vi "Teleop.vi"(10 "Match Info":T1={"Autonomous Elapsed Seconds"=0.0, "TeleOp Elapsed Seconds"=0.0, "Disabled Elapsed Seconds"=0.0, "Visited Autonomous"=FALSE, "Visited TeleOp"=FALSE, "Visited Disabled"=FALSE, "Autonomous Settings"={"Autonomous Style"=enum."Independent", "VI Refnum"=refnum}}, 11 "Call Context":T2) -> ()   [LabVIEW 2019]
doc: "This VI is called for each enabled TeleOp packet received from the DS. It is typically used to read from joysticks and other inputs and update I/O or setpoints for timed control loops. It should complete and return within 20 milliseconds or risk missing DS packets."
uses:
  <vilib>/Rock Robotics/WPI/DriverStation/WPI_DriverStationDerivedRobotMode.ctl
  <vilib>/Rock Robotics/WPI/DriverStation/WPI_DriverStationMatch Info.ctl
  Framework/Robot Global Data.vi
  <vilib>/Rock Robotics/Network Tables/NT Write Boolean.vi
  <vilib>/Rock Robotics/Network Tables/NT Write Number.vi
  <vilib>/Rock Robotics/Network Tables/NT Write Numeric Array.vi
  <vilib>/Rock Robotics/Network Tables/NT Write Boolean Array.vi
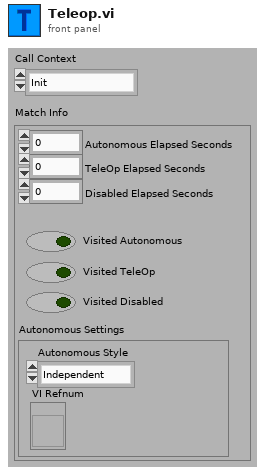
[diagram p1: front panel]
types:
  T1 = typedef "WPI_DriverStationMatch Info.ctl" = cluster{"Autonomous Elapsed Seconds":dbl, "TeleOp Elapsed Seconds":dbl, "Disabled Elapsed Seconds":dbl, "Visited Autonomous":bool, "Visited TeleOp":bool, "Visited Disabled":bool, "Autonomous Settings":cluster{"Autonomous Style":enum16{"Iterative", "Independent"}, "VI Refnum":refnum<vi>}}
  T2 = typedef "WPI_DriverStationDerivedRobotMode.ctl" = enum16{"Init", "Execute", "Stop"}
  T3 = typedef "WPI_JoystickDevRef.ctl" = cluster{"Device":T4}
  T4 = typedef "WPI_JoystickDeviceEnum.ctl" = enum16{"USB 0", "USB 1", "USB 2", "USB 3", "USB 4", "USB 5"}
  T5 = typedef "Command Status Info.ctl" = cluster{"Name":string, "Status":T6, "notifier out":T7}
  T6 = typedef "Completion Status.ctl" = enum16{"Successful", "Aborted", "Incomplete"}
  T7 = typedef "Completion Notifier.ctl" = refnum<notifier>
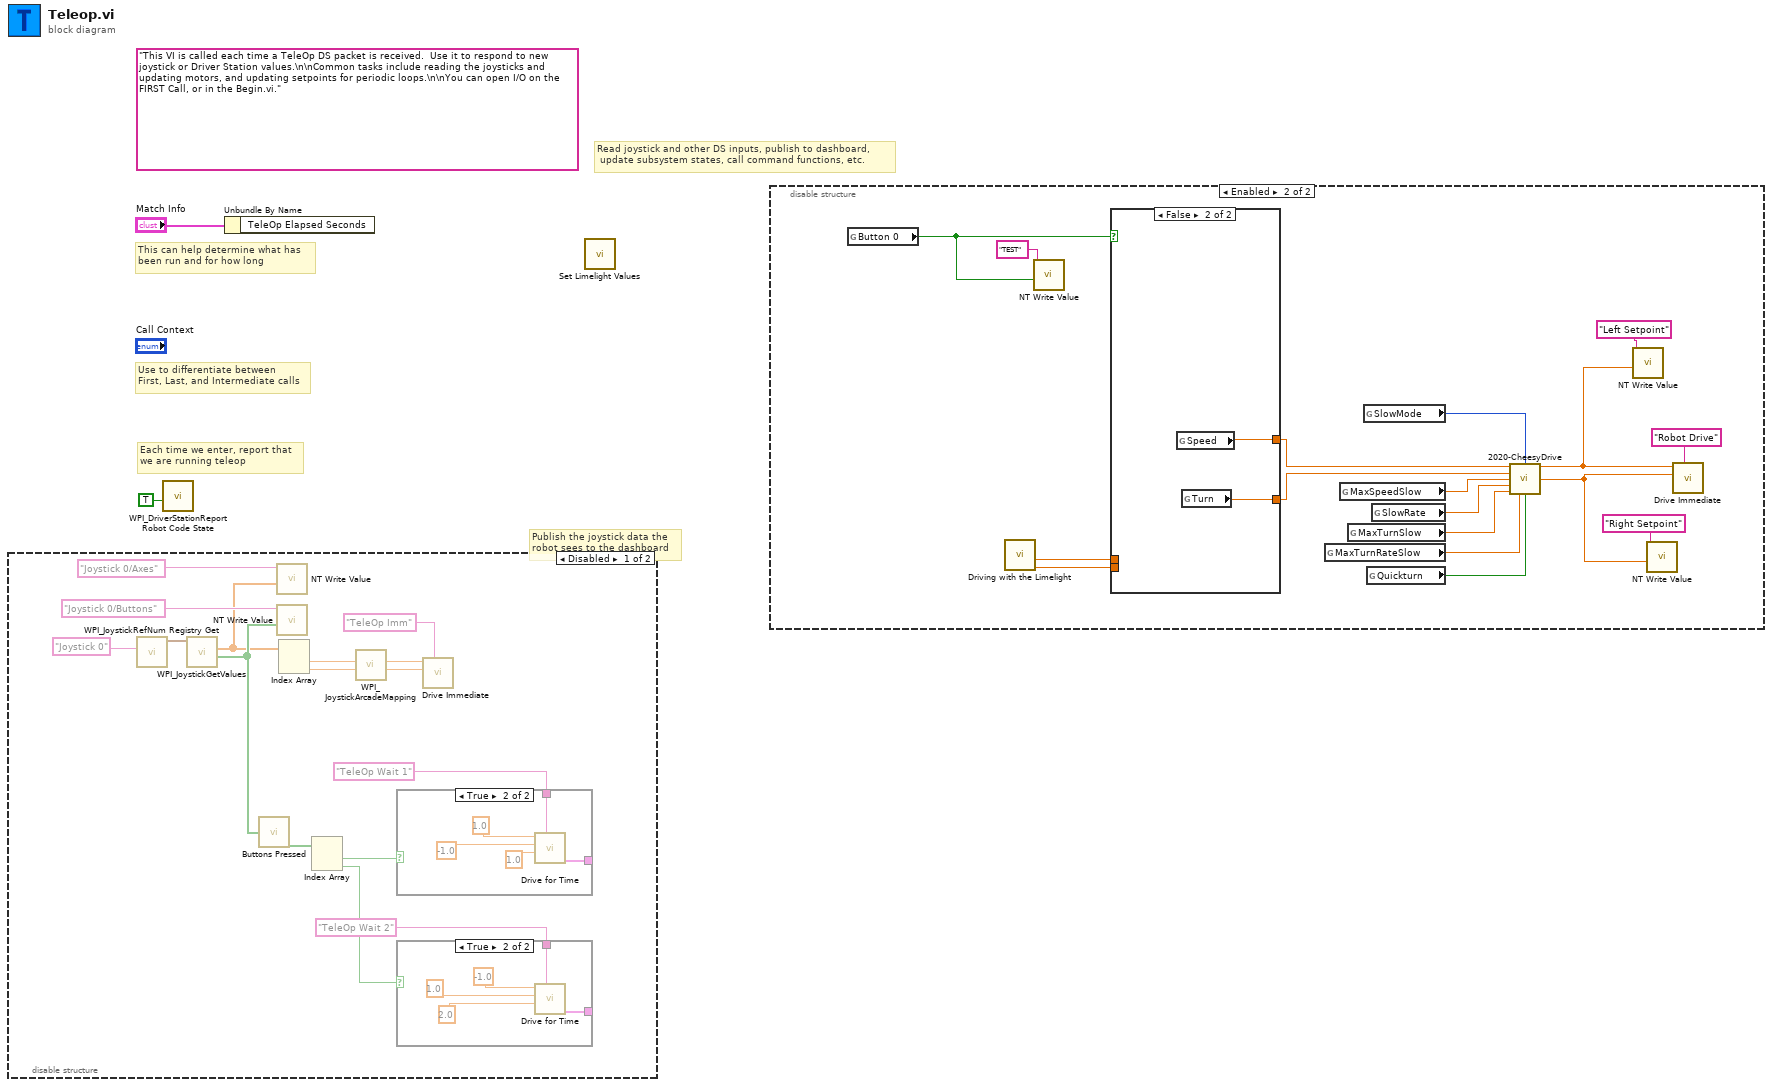
[diagram p0: block diagram]
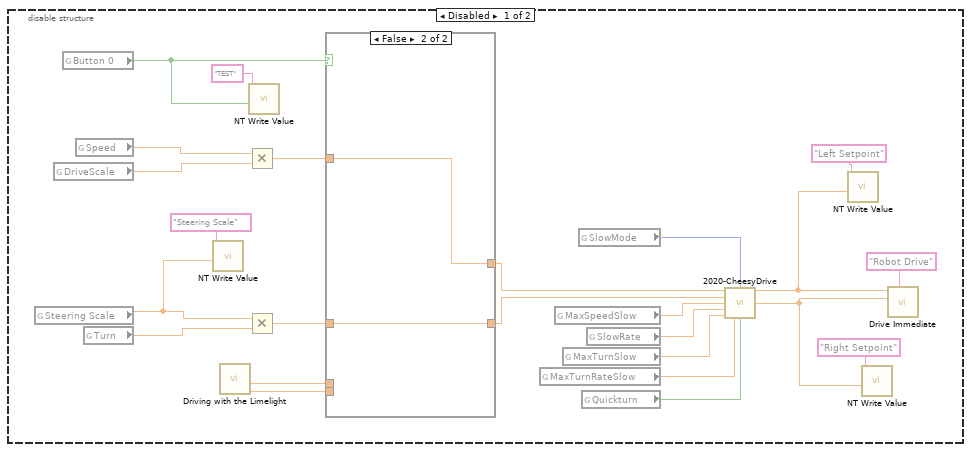
[diagram p2: hidden frame]
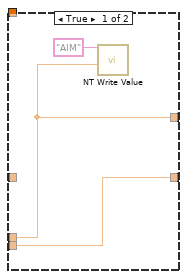
[diagram p3: hidden frame]
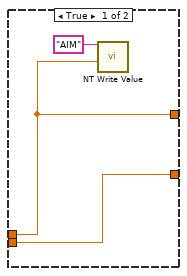
[diagram p4: hidden frame]
diagram:
  (unwired) "This VI is called each time a TeleOp DS packet is received.  Use it to respond to new joystick or Driver Station values.\n\nCommon tasks include reading the joysticks and updating motors, and updating setpoints for periodic loops.\n\nYou can open I/O on the FIRST Call, or in the Begin.vi."
  # "Publish the joystick data the\nrobot sees to the dashboard"
  # "Read joystick and other DS inputs, publish to dashboard,\n update subsystem states, call command functions, etc."
  # "Each time we enter, report that\nwe are running teleop"
  # "Use to differentiate between\nFirst, Last, and Intermediate calls"
  # "This can help determine what has\nbeen run and for how long"
  n1 = disable-structure shown="Disabled" {
    frame Disabled {
      n2 = call <vilib>:"WPI_JoystickRefNum Registry Get.vi"("refnum name"="Joystick 0") -> ("JoystickDevRef"=w17:T3)  [unwired: 1 in, 9 out]
      n3 = call <vilib>:"WPI_JoystickGetValues.vi"("JoystickDevRef"=w17) -> ("Buttons"=w5:bool[], "Axes"=w4:dbl[])  [unwired: 6 in, 3 out]
      n4 = call "Buttons Pressed.vi"("Button Values"=w5) -> ("Button Presses"=w13:bool[])
      n5 = call-poly <vilib>:"NT Write Value.vi"("Numeric Array"=w4, "Name"="Joystick 0/Axes") -> ()  [unwired: 9 in, 1 out]
      n6 = call-poly <vilib>:"NT Write Value.vi"("Boolean Array"=w5, "Name"="Joystick 0/Buttons") -> ()  [unwired: 9 in, 1 out]
      n7 = Index Array(array=w4) -> (element #1=w8:dbl, element #2=w7:dbl)  [unwired: 2 in]
      n8 = Index Array(array=w13) -> (element #1=w12:bool, element #2=w11:bool)  [unwired: 2 in]
      n9 = call <vilib>:"WPI_JoystickArcadeMapping.vi"("Y axis value"=w7, "X axis value"=w8) -> ("Right Motor Value"=w9:dbl, "Left Motor Value"=w10:dbl)  [unwired: 8 in]
      n10 = case shown="True" w12 {
        tunnel: [_ w27] -> _
        tunnel: "TeleOp Wait 1" ("Description") -> [_ w26]
        frame False {
        }
        frame True {
          n11 = call "Drive for Time.vi"("Description"=w26, "Seconds"=1.0, "Right Speed"=-1.0, "Left Speed"=1.0) -> ("Command Info Out"=w27:T5)  [unwired: 7 in]
        }
      }
      n12 = case shown="True" w11 {
        tunnel: [_ w21] -> _
        tunnel: "TeleOp Wait 2" ("Description") -> [_ w20]
        frame False {
        }
        frame True {
          n13 = call "Drive for Time.vi"("Description"=w20, "Seconds"=2.0, "Right Speed"=1.0, "Left Speed"=-1.0) -> ("Command Info Out"=w21:T5)  [unwired: 7 in]
        }
      }
      n14 = call "Drive Immediate.vi"("Description"="TeleOp Imm", "Right Setpoint"=w9, "Left Setpoint"=w10) -> ()  [unwired: 8 in, 1 out]
    }
    frame Enabled {
    }
  }
  n15 = call <vilib>:"WPI_DriverStationReport Robot Code State.vi"("TeleOp"=TRUE ("Autonomous")) -> ()  [unwired: 10 in, 1 out]
  n16 = Unbundle By Name("Match Info") -> ()  [unwired: 1 out]
  n17 = call "Set Limelight Values.vi"() -> ()  [unwired: 12 in]
  n18 = disable-structure shown="Enabled" {
    frame Disabled {
      n19 = global read "Robot Global Data.vi" "Steering Scale"() -> (w30:dbl)
      n20 = global read "Robot Global Data.vi" "DriveScale"() -> (w29:dbl)
      n21 = global read "Robot Global Data.vi" "Button 0"() -> (w39:bool)
      n22 = global read "Robot Global Data.vi" "Speed"() -> (w40:dbl)
      n23 = global read "Robot Global Data.vi" "Turn"() -> (w41:dbl)
      n24 = call-poly <vilib>:"NT Write Value.vi"("Numeric"=w30, "Name"="Steering Scale") -> ()  [unwired: 9 in, 1 out]
      n25 = call "Driving with the Limelight.vi"() -> ("TurnCommand"=w45:dbl, "SpeedCommand"=w44:dbl)  [unwired: 9 in, 1 out]
      n26 = Multiply(x=w40, y=w29) -> (x*y=w50:dbl)
      n27 = Multiply(x=w30, y=w41) -> (x*y=w51:dbl)
      n28 = call-poly <vilib>:"NT Write Value.vi"("Boolean"=w39, "Name"="TEST") -> ()  [unwired: 9 in, 1 out]
      n29 = case shown="False" w39 {
        tunnel: w51 -> [_ w57]
        tunnel: w50 -> [_ w56]
        tunnel: [w54 w56] -> w48
        tunnel: w45 -> [w53 _]
        tunnel: w44 -> [w54 _]
        tunnel: [w53 w57] -> w42
        frame True {
          n30 = call-poly <vilib>:"NT Write Value.vi"("Numeric"=w54, "Name"="AIM") -> ()  [unwired: 9 in, 1 out]
        }
        frame False {
        }
      }
      n31 = global read "Robot Global Data.vi" "MaxTurnRateSlow"() -> (w31:dbl)
      n32 = global read "Robot Global Data.vi" "MaxSpeedSlow"() -> (w34:dbl)
      n33 = global read "Robot Global Data.vi" "MaxTurnSlow"() -> (w32:dbl)
      n34 = global read "Robot Global Data.vi" "SlowMode"() -> (w47:u32)
      n35 = global read "Robot Global Data.vi" "Quickturn"() -> (w43:bool)
      n36 = global read "Robot Global Data.vi" "SlowRate"() -> (w33:dbl)
      n37 = call "2020-CheesyDrive.vi"("Throttle"=w48, "SlowMode"=w47, "Wheel"=w42, "MaxSpeedSlow"=w34, "SlowRate"=w33, "MaxTurnSlow"=w32, "MaxTurnRateSlow"=w31, "Quickturn"=w43) -> ("Left PWM"=w36:dbl, "Right PWM"=w35:dbl)  [unwired: 6 in]
      n38 = call-poly <vilib>:"NT Write Value.vi"("Numeric"=w36, "Name"="Left Setpoint") -> ()  [unwired: 9 in, 1 out]
      n39 = call-poly <vilib>:"NT Write Value.vi"("Numeric"=w35, "Name"="Right Setpoint") -> ()  [unwired: 9 in, 1 out]
      n40 = call "Drive Immediate.vi"("Description"="Robot Drive", "Right Setpoint"=w35, "Left Setpoint"=w36) -> ()  [unwired: 8 in, 1 out]
    }
    frame Enabled {
      n41 = global read "Robot Global Data.vi" "Button 0"() -> (w66:bool)
      n42 = call "Driving with the Limelight.vi"() -> ("TurnCommand"=w70:dbl, "SpeedCommand"=w69:dbl)  [unwired: 9 in, 1 out]
      n43 = call-poly <vilib>:"NT Write Value.vi"("Boolean"=w66, "Name"="TEST") -> ()  [unwired: 9 in, 1 out]
      n44 = case shown="False" w66 {
        tunnel: [w76 w79] -> w73
        tunnel: w70 -> [w75 _]
        tunnel: w69 -> [w76 _]
        tunnel: [w75 w78] -> w67
        frame True {
          n45 = call-poly <vilib>:"NT Write Value.vi"("Numeric"=w76, "Name"="AIM") -> ()  [unwired: 9 in, 1 out]
        }
        frame False {
          n46 = global read "Robot Global Data.vi" "Speed"() -> (w79:dbl)
          n47 = global read "Robot Global Data.vi" "Turn"() -> (w78:dbl)
        }
      }
      n48 = global read "Robot Global Data.vi" "MaxTurnRateSlow"() -> (w58:dbl)
      n49 = global read "Robot Global Data.vi" "MaxSpeedSlow"() -> (w61:dbl)
      n50 = global read "Robot Global Data.vi" "MaxTurnSlow"() -> (w59:dbl)
      n51 = global read "Robot Global Data.vi" "SlowMode"() -> (w72:u32)
      n52 = global read "Robot Global Data.vi" "Quickturn"() -> (w68:bool)
      n53 = global read "Robot Global Data.vi" "SlowRate"() -> (w60:dbl)
      n54 = call "2020-CheesyDrive.vi"("Throttle"=w73, "SlowMode"=w72, "Wheel"=w67, "MaxSpeedSlow"=w61, "SlowRate"=w60, "MaxTurnSlow"=w59, "MaxTurnRateSlow"=w58, "Quickturn"=w68) -> ("Left PWM"=w63:dbl, "Right PWM"=w62:dbl)  [unwired: 6 in]
      n55 = call-poly <vilib>:"NT Write Value.vi"("Numeric"=w63, "Name"="Left Setpoint") -> ()  [unwired: 9 in, 1 out]
      n56 = call-poly <vilib>:"NT Write Value.vi"("Numeric"=w62, "Name"="Right Setpoint") -> ()  [unwired: 9 in, 1 out]
      n57 = call "Drive Immediate.vi"("Description"="Robot Drive", "Right Setpoint"=w62, "Left Setpoint"=w63) -> ()  [unwired: 8 in, 1 out]
    }
  }
